vi "Remove UUID Contact.vi"(8 "error in (no error)":errorcluster, 11 "UUID":string) -> (0 "error out":errorcluster)   [LabVIEW 2014, in "Contact Data.lvlib"]
doc: "Removes a contact from the address book data store."
uses:
  Contact Data.lvlib
  Command.ctl
  Contact.ctl
  Position.ctl
  Controls.ctl
  DestinationCluster.ctl
  DesinationControls.ctl
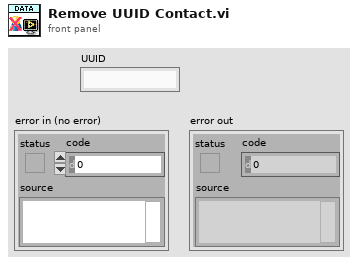
[diagram p1: front panel]
types:
  T1 = typedef "Contact Data.lvlib/Contact.ctl" = cluster{"ID":u32, "UUID":string, "Name":string, "Iteration":i32, "Posit Array":T2[], "Controls":T3, "DestArray":T4[], "SetSpeed":dbl, "Speed":dbl}
  T2 = typedef "Contact Data.lvlib/Position.ctl" = cluster{"X":dbl, "Y":dbl, "Z":dbl}
  T3 = typedef "Contact Data.lvlib/Controls.ctl" = cluster{"throttle":dbl, "brake":dbl, "horn":dbl, "wait":dbl}
  T4 = typedef "Contact Data.lvlib/DestinationCluster.ctl" = cluster{"Desination":string, "DestControls":T5, "Timer":u32, "Set Timer":u32, "Time Stamp":timestamp, "Repeat?":bool, "Optional Data":string, "Distance":dbl}
  T5 = typedef "Contact Data.lvlib/DesinationControls.ctl" = enum16{"Tracker", "Manual", "Stop", "Station DateTime", "Station Timer", "Maintain"}
  T6 = typedef "Contact Data.lvlib/Command.ctl" = enum16{"Set All Contacts", "Load", "Save", "Get All Data", "Get Single Data (ID)", "Get Single Data", "Set Position", "Set Destinations", "Set Controls", "Remove Single Data", "Remove UUID Contact", "Set Single ALL", "Is Data Modified", "Import Data"}
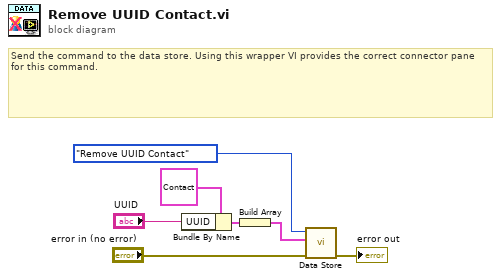
[diagram p0: block diagram]
diagram:
  # "Send the command to the data store. Using this wrapper VI provides the correct connector pane for this command."
  n1 = Bundle By Name(cluster=T1 {"ID"=0, "UUID"="", "Name"="", "Iteration"=0, "Posit Array"=[], "Controls"={"throttle"=0.0, "brake"=0.0, "horn"=0.0, "wait"=0.5}, "DestArray"=[], "SetSpeed"=0.0, "Speed"=0.0} ("Contact"), "UUID"="UUID") -> (w5:T1)
  n2 = Build Array(w5) -> (w2:T1[])
  n3 = call "Data Store.vi"("error in (no error)"="error in (no error)", "Contact in"=w2, "Command"=Command."Remove UUID Contact") -> ("error out"=→"error out":errorcluster)  [unwired: 6 in, 2 out]
